vi "FRC Color Processing Example.vi"() -> ()   [LabVIEW 2015]
uses:
  <vilib>/Rock Robotics/WPI/Camera/WPI_CameraSettings Read MJPG.ctl
  <vilib>/Rock Robotics/WPI/Camera/WPI_CameraImageSize.ctl
  Vision Support Code/Camera Types.ctl
  <vilib>/vision/NI_Vision_Development_Module.lvlib
panel:
  in  "Std Devs for Calibration":cluster{"H":dbl, "S":dbl, "V":dbl}={"H"=4.0, "S"=6.0, "V"=6.0}
  out "Highest Avg Score":dbl format="%#_3g"
  in  "Min Score Threshold":i32=70
  in  "Emphasize Limit Tests":bool=TRUE
  in  "Camera Type":T1=enum."MS HD3000 square"
  in  "image files":string[](array[string])
  in  "Aspect Ratio Fudge Factor":dbl=1.0
  out "Detected Targets":T2(array[cluster]) {"Normalized Rect"."Numeric 5" format="%#_2g"; "Normalized Rect"."Numeric 3" format="%#_2g"; "Normalized Rect"."Numeric 2" format="%#_2g"; "Normalized Rect"."Numeric" format="%#_2g"}
  in  "Annotation Limit":dbl=75.0
  in  "Source":enum32{"Files", "Camera"}(tab)
  in  "Images":i32(listbox)
  in  "Folder Location":path=path "C:/Program Files (x86)/National Instruments/LabVIEW 2015/examples/FRC/roboRIO/Vision/2016 Vision Example/Sample Images/Real Tower"
  in  "Camera Settings":T3={"fps"=20, "compression"=30, "Image Size"=enum."320x240"}
  in  "Camera Address":string="USB 1"
  in  "Annotate":bool=TRUE
  out "Sorted Particle Scores":T5(array[cluster]) {"Moment Factor" format="%#_3g"; "Aspect Ratio" format="%#_3g"; "Area to CH" format="%#_3g"; "X" format="%#_3g"; "Y" format="%#_3g"}
  out "Qualified Particles":i32
  in  "LED Color":T6={"Hue"={110.52399131877658, 148.6727294921875}, "Sat"={34.78571428571429, 255.0}, "Val"={91.07142857142858, 255.0}} {"Hue" scale=0.0..255.0 scale format="%#_3g"}
  out "Masked":T7(plugin-control)
  out "Original Image":T7(plugin-control)
  # "Instructions:\nUse Source to select image files from a directory, or use a USB or IP camera connected to your laptop.\nUse LED Color to threshold and build particles. Adjust HSV values to improve masking.\nClick and draw a line in Original Image to auto-calibrate to the LED color. You may need to widen Sat and Val.\nAnnotations draw a rectangle around \"good\" particles with scores from top to bottom."
  # "Density Profile"
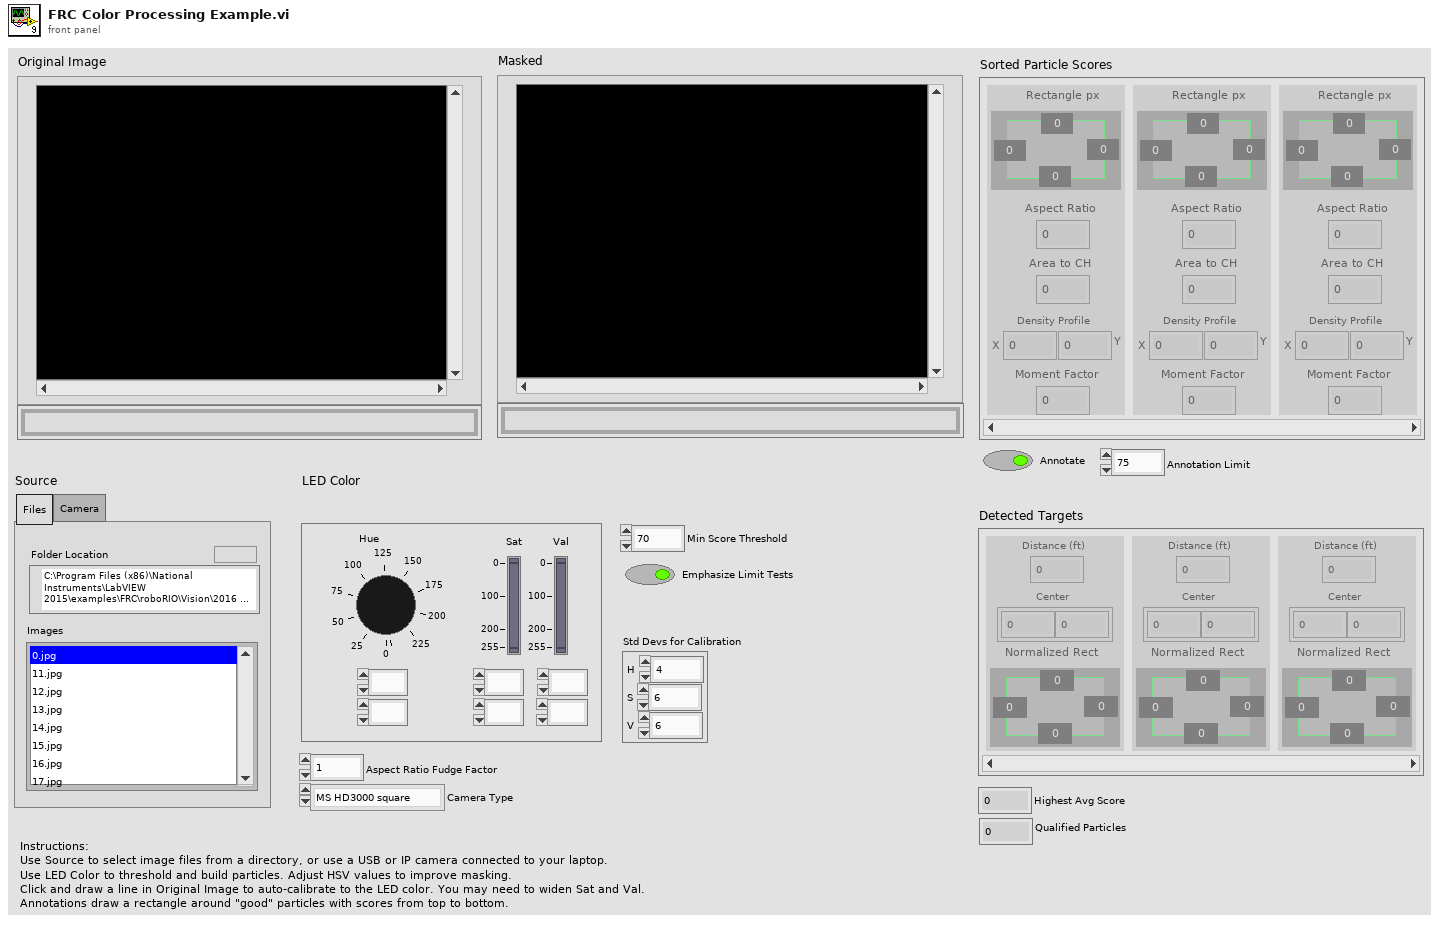
[diagram p1: front panel]
types:
  T1 = typedef "Camera Types.ctl" = enum16{"206", "1011", "1013", "MS HD3000 square", "MS HD3000 640x480"}
  T2 = cluster{"Distance (ft)":dbl, "Center":cluster{dbl, dbl}, "Normalized Rect":cluster{"Numeric":dbl, "Numeric 2":dbl, "Numeric 3":dbl, "Numeric 5":dbl}}[]
  T3 = typedef "WPI_CameraSettings Read MJPG.ctl" = cluster{"fps":i32, "compression":i32, "Image Size":T4}
  T4 = typedef "WPI_CameraImageSize.ctl" = enum16{"640x480", "320x240", "160x120", "Custom"}
  T5 = cluster{"Rectangle px":cluster{"Numeric":dbl, "Numeric 2":dbl, "Numeric 3":dbl, "Numeric 5":dbl}, "Aspect Ratio":dbl, "Area to CH":dbl, "X":dbl, "Y":dbl, "Moment Factor":dbl}[]
  T6 = cluster{"Hue":cluster{dbl, dbl}, "Sat":cluster{dbl, dbl}, "Val":cluster{dbl, dbl}}
  T7 = typedef "IMAQ Image.ctl" = refnum<image>
  T8 = typedef "Particle Parameters" = i32
  T9 = typedef "Image Type" = u32
  T10 = cluster{cluster{dbl, dbl}, cluster{dbl, dbl}, cluster{dbl, dbl}}
  T11 = cluster{"Bounding box":cluster{"left":dbl, "top":dbl, "right":dbl, "bottom":dbl}, "Aspect Ratio":dbl, "Area to CH":dbl, "X Mask":dbl, "Y Mask":dbl, "Moment":dbl}[]
  T12 = cluster{"Rectangle":cluster{"Numeric":dbl, "Numeric 2":dbl, "Numeric 3":dbl, "Numeric 5":dbl}, "L":dbl, "Area to CH":dbl, "X":dbl, "Y":dbl, "Moment Factor":dbl}[]
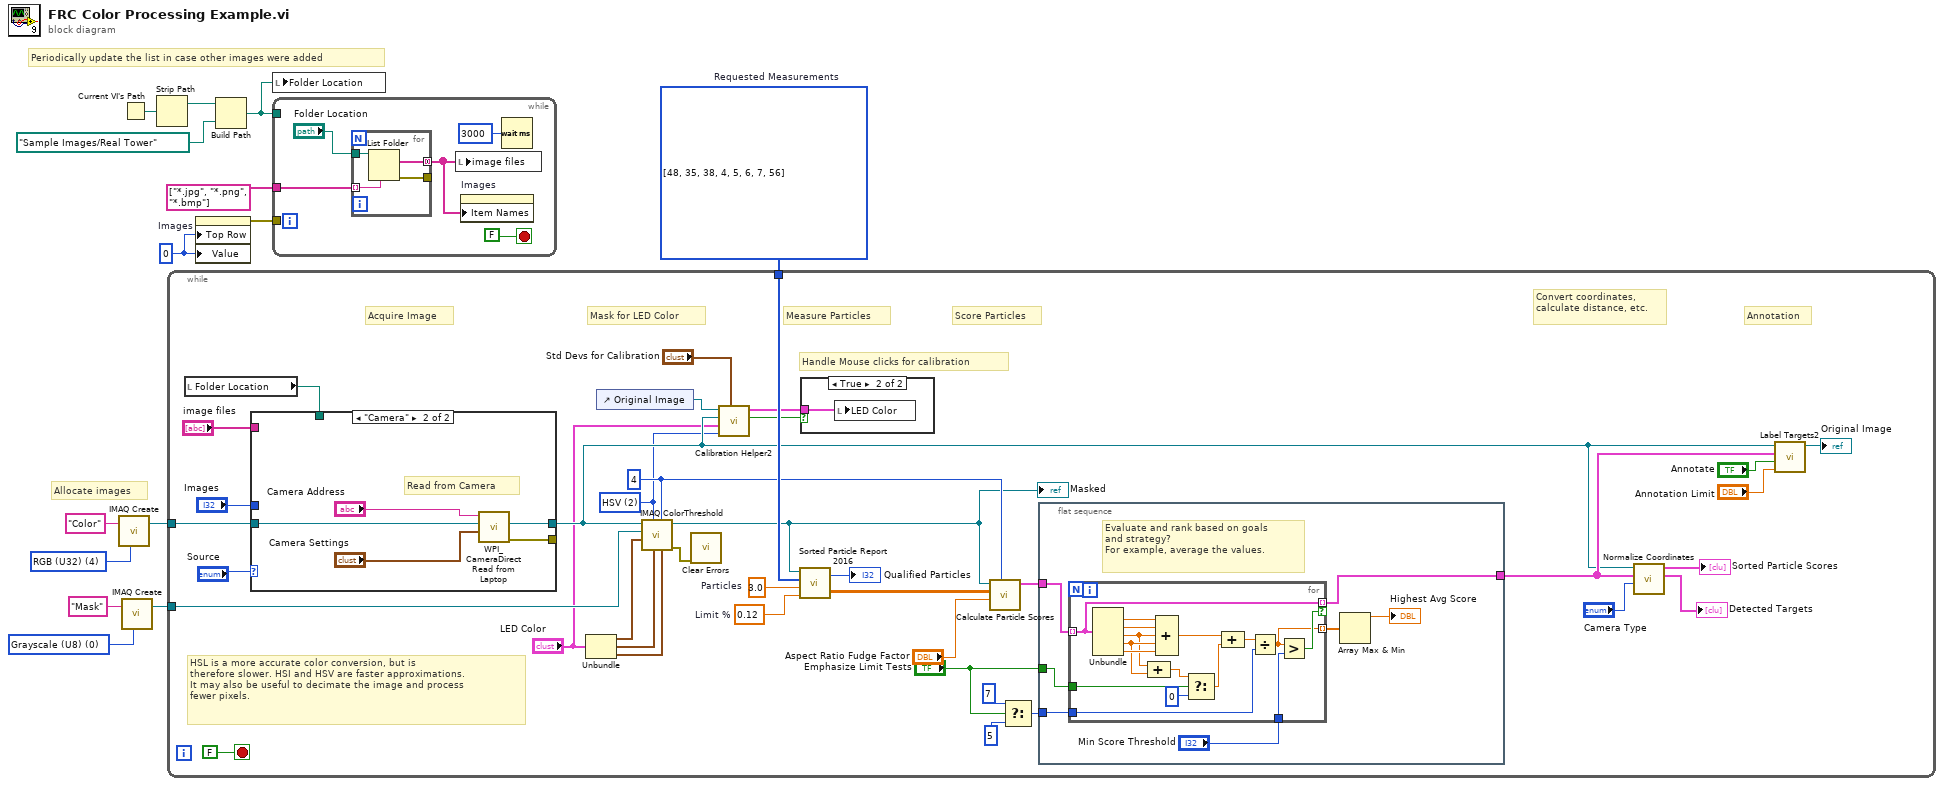
[diagram p0: block diagram]
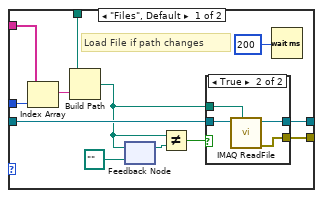
[diagram p3: hidden frame]
diagram:
  w2 = u32 0 ("milliseconds to wait")
  w8 = T8[] [48, 35, 38, 4, 5, 6, 7, 56] items=["Center of Mass X", "Center of Mass Y", "First Pixel X", "First Pixel Y", "Bounding Rect Left", "Bounding Rect Top", "Bounding Rect Right", "Bounding Rect Bottom", "Max Feret Diameter Start X", "Max Feret Diameter Start Y", "Max Feret Diameter End X", "Max Feret Diameter End Y", "Max Horiz. Segment Length Left", "Max Horiz. Segment Length Right", "Max Horiz. Segment Length Row", "-", "Bounding Rect Width", "Bounding Rect Height", "Bounding Rect Diagonal", "Perimeter", "Convex Hull Perimeter", "Holes' Perimeter", "Max Feret Diameter", "Equivalent Ellipse Major Axis", "Equivalent Ellipse Minor Axis", "Equivalent Ellipse Minor Axis (Feret)", "Equivalent Rect Long Side", "Equivalent Rect Short Side", "Equivalent Rect Diagonal", "Equivalent Rect Short Side (Feret)", "Average Horiz. Segment Length", "Average Vert. Segment Length", "Hydraulic Radius", "Waddel Disk Diameter", "-", "Area", "Holes' Area", "Particle & Holes' Area", "Convex Hull Area", "Image Area", "-", "Number of Holes", "Number of Horiz. Segments", "Number of Vert. Segments", "-", "Orientation", "Max Feret Diameter Orientation", "-", "% Area/Image Area", "% Area/(Particle & Holes' Area)", "Ratio of Equivalent Ellipse Axes", "Ratio of Equivalent Rect Sides", "-", "Elongation Factor", "Compactness Factor", "Heywood Circularity Factor", "Type Factor", "-", "Sum X", "Sum Y", "Sum XX", "Sum XY", "Sum YY", "Sum XXX", "Sum XXY", "Sum XYY", "Sum YYY", "-", "Moment of Inertia XX", "Moment of Inertia XY", "Moment of Inertia YY", "Moment of Inertia XXX", "Moment of Inertia XXY", "Moment of Inertia XYY", "Moment of Inertia YYY", "Norm. Moment of Inertia XX", "Norm. Moment of Inertia XY", "Norm. Moment of Inertia YY", "Norm. Moment of Inertia XXX", "Norm. Moment of Inertia XXY", "Norm. Moment of Inertia XYY", "Norm. Moment of Inertia YYY", "Hu Moment 1", "Hu Moment 2", "Hu Moment 3", "Hu Moment 4", "Hu Moment 5", "Hu Moment 6", "Hu Moment 7"]  # Requested Measurements
  w11 = T9 0 items=["Grayscale (U8)", "Grayscale (I16)", "Grayscale (SGL)", "Complex (CSG)", "RGB (U32)", "HSL (U32)", "RGB (U64)", "Grayscale (U16)"] ("Image Type")
  w13 = T9 4 items=["Grayscale (U8)", "Grayscale (I16)", "Grayscale (SGL)", "Complex (CSG)", "RGB (U32)", "HSL (U32)", "RGB (U64)", "Grayscale (U16)"] ("Image Type")
  # "Periodically update the list in case other images were added"
  # "Allocate images"
  n1 = call "IMAQ Create"("Image Name"="Color", "Image Type"=w13) -> ("New Image"=w12:T7)  [unwired: 2 in, 2 out]
  n2 = Current VI's Path() -> (path=w7:path)
  n3 = call "IMAQ Create"("Image Name"="Mask", "Image Type"=w11) -> ("New Image"=w9:T7)  [unwired: 2 in, 2 out]
  n4 = Strip Path(path=w7) -> (stripped path=w5:path)  [unwired: 1 out]
  n5 = while {
    tunnel: w12 -> [w51]
    tunnel: w9 -> [w49]
    tunnel: w8 -> [w45]
    stop <- FALSE stop-if-true
    w37 = 4 ("Replace Value")
    w41 = 0.12  # Limit %
    w44 = 3.0  # Particles
    w19 = u16 2 items=["RGB", "HSL", "HSV", "HSI"] ("Color Mode")
    # "Handle Mouse clicks for calibration"
    # "Measure Particles"
    # "Convert coordinates,\ncalculate distance, etc."
    # "Annotation"
    # "Score Particles"
    # "Mask for LED Color"
    # "Acquire Image"
    # "HSL is a more accurate color conversion, but is\ntherefore slower. HSI and HSV are faster approximations.\nIt may also be useful to decimate the image and process\nfewer pixels."
    n6 = local read "Folder Location"() -> (w16:path)
    n7 = case shown="\"Camera\"" "Source" {
      tunnel: [w87 w98] -> _
      tunnel: [w88 w97] -> w22
      tunnel: w51 -> [w86 w96]
      tunnel: "image files" -> [w78 _]
      tunnel: "Images" -> [w85 _]
      tunnel: w16 -> [w83 _]
      frame "Files", Default {
        # "Load File if path changes"
        n8 = Index Array(array=w78, index=w85) -> (element=w84:string)
        n9 = Build Path(base path=w83, name or relative path=w84) -> (appended path=w79:path)
        n10 = feedback-in #1(w79) -> ()
        n11 = feedback #1(path "" ("appended path")) -> (w81:path)
        n12 = Not Equal?(x=w79, y=w81) -> (x != y?=w82:bool)
        n13 = case shown="True" w82 {
          tunnel: [w89 w93] -> w88
          tunnel: [_ w92] -> w87
          tunnel: w86 -> [w89 w91]
          tunnel: w79 -> [_ w90]
          frame False {
          }
          frame True {
            n14 = call "IMAQ ReadFile"("File Path"=w90, "Image"=w91) -> ("error out"=w92:errorcluster, "Image Out"=w93:T7)  [unwired: 5 in, 3 out]
          }
        }
        n15 = Wait (ms)(milliseconds to wait=u32 200 ("delay (ms)")) -> ()  [unwired: 1 out]
      }
      frame "Camera" {
        # "Read from Camera"
        n16 = call <vilib>:"WPI_CameraDirect Read from Laptop.vi"("Camera Settings"="Camera Settings", "Image"=w96, "address"="Camera Address") -> ("error out"=w98:errorcluster, "Image Out"=w97:T7)  [unwired: 7 in]
      }
    }
    n17 = Unbundle("LED Color") -> ("Hue"=w48:cluster{dbl, dbl}, "Sat"=w47:cluster{dbl, dbl}, "Val"=w46:cluster{dbl, dbl})
    n18 = control-ref of="Original Image"() -> (w23:refnum<vi>)
    n19 = call "IMAQ ColorThreshold"("Blue or Luma or Val or Inten Range"=w46, "Replace Value"=w37, "Green or Sat Range"=w47, "Color Mode"=w19, "Red or Hue Range"=w48, "Image Dst"=w49, "Image Src"=w22) -> ("error out"=w27:errorcluster, "Image Dst Out"=w28:T7)  [unwired: 3 in]
    "Masked" <- w28
    n20 = call <vilib>:"Clear Errors.vi"("error in (no error)"=w27) -> ()  [unwired: 5 in, 2 out]
    n21 = call "Calibration Helper2.vi"("Std Devs"="Std Devs for Calibration", "Color Mode"=w19, "Color Components"="LED Color", "Image"=w22, "Image Ctl Refnum"=w23) -> ("Changed"=w21:bool, "output color"=w20:T10)  [unwired: 5 in]
    n22 = call "Sorted Particle Report 2016.vi"("Min Area Size %"=w41, "Particle Count Limit"=w44, "Pixel Measurements"=w45, "Image in"=w28) -> ("Sorted Data"=w42:dbl[][], "Particles"=→"Qualified Particles":i32)
    n23 = case shown="True" w21 {
      tunnel: w20 -> [_ w53]
      frame False {
      }
      frame True {
        n24 = local write "LED Color"(w53) -> ()
      }
    }
    n25 = call "Calculate Particle Scores.vi"("Pixel Value"=w37, "Aspect Fudge Factor"="Aspect Ratio Fudge Factor", "Sorted Data"=w42, "Image in"=w28) -> ("Scores"=w31:T11)  [unwired: 7 in]
    n26 = Select(t=7, s="Emphasize Limit Tests", f=5) -> (s? t:f=w24:i32)
    n27 = flat-sequence {
      tunnel: w31 -> [w59]
      tunnel: [w60] -> w29
      tunnel: w24 -> [w56]
      tunnel: "Emphasize Limit Tests" -> [w54]
      frame #0 {
        # "Evaluate and rank based on goals\nand strategy?\nFor example, average the values."
        n28 = for {
          tunnel: w59 -> [w74] mode=indexing
          tunnel: [w74] -> w60 mode=indexing if=w73
          tunnel: [w72] -> w58 mode=indexing
          tunnel: w56 -> [w71]
          tunnel: "Min Score Threshold" -> [w70]
          tunnel: w54 -> [w63]
          n29 = Unbundle(w74) -> ("Aspect Ratio"=w76:dbl, "Area to CH"=w75:dbl, "X Mask"=w65:dbl, "Y Mask"=w66:dbl, "Moment"=w67:dbl)  [unwired: 1 out]
          n30 = Compound Arithmetic op=ADD(w65, w66) -> (w64:dbl)
          n31 = Compound Arithmetic op=ADD(w76, w75, w65, w66, w67) -> (w69:dbl)
          n32 = Select(t=w64, s=w63, f=0) -> (s? t:f=w62:dbl)
          n33 = Compound Arithmetic op=ADD(w69, w62) -> (w68:dbl)
          n34 = Divide(x=w68, y=w71) -> (x/y=w72:dbl)
          n35 = Greater?(x=w72, y=w70) -> (0:w73:bool)
        }
        n36 = Array Max & Min(array=w58) -> (max value=→"Highest Avg Score":dbl)  [unwired: 3 out]
      }
    }
    n37 = call "Normalize Coordinates.vi"("Camera Type"="Camera Type", "Targets"=w29, "Image in"=w22) -> ("Found Targets"=→"Detected Targets":T2, "Sorted Scores"=→"Sorted Particle Scores":T12)  [unwired: 7 in]
    n38 = call "Label Targets2.vi"("Score Threshold"="Annotation Limit", "Annotate"="Annotate", "Targets"=w29, "Image in"=w22) -> ("Image out"=→"Original Image":T7)  [unwired: 7 in]
  }
  n39 = property on="Images" class="LstBox (strict)"("Top Row"=w2, "Value"=w2) -> (error out=w3:errorcluster)  [unwired: 2 in, 1 out]
  n40 = Build Path(base path=w5, name or relative path=path "Sample Images/Real Tower" ("Folder Location")) -> (appended path=w4:path)
  n41 = local write "Folder Location"(w4) -> ()
  n42 = while {
    tunnel: w4 -> [_]
    tunnel: w3 -> [_]
    tunnel: string[] ["*.jpg", "*.png", "*.bmp"] -> [w99]
    stop <- FALSE stop-if-true
    n43 = for {
      tunnel: [w107] -> w101 mode=concatenating
      tunnel: "Folder Location" -> [w106]
      tunnel: [w105] -> _
      tunnel: w99 -> [w104] mode=indexing
      n44 = List Folder(path=w106, pattern=w104) -> (filenames=w107:string[], error out=w105:errorcluster)  [unwired: 2 in, 2 out]
    }
    n45 = local write "image files"(w101) -> ()
    n46 = property on="Images" class="LstBox (strict)"("Item Names"=w101) -> ()  [unwired: 2 in, 2 out]
    n47 = Wait (ms)(milliseconds to wait=u32 3000) -> ()  [unwired: 1 out]
  }
